vi "GVar.vi"(6 "Action":T3, 11 "Parameters In":T1={"Stop"=FALSE, "Play"=FALSE, "number of samples/ch"=12000, "sound format"={"sample rate (S/s)"=48000.0, "number of channels"=2, "bits per sample"=24}, "Path"=path ""}) -> (3 "Parameters In 2":T1={"Stop"=FALSE, "Play"=FALSE, "number of samples/ch"=12000, "sound format"={"sample rate (S/s)"=48000.0, "number of channels"=2, "bits per sample"=24}, "Path"=path ""})   [LabVIEW 2023]
uses:
  <vilib>/sound2/lvsound2.llb/Sound Data Format.ctl
  Controls/Enum 1.ctl
  Controls/Parameters In.ctl
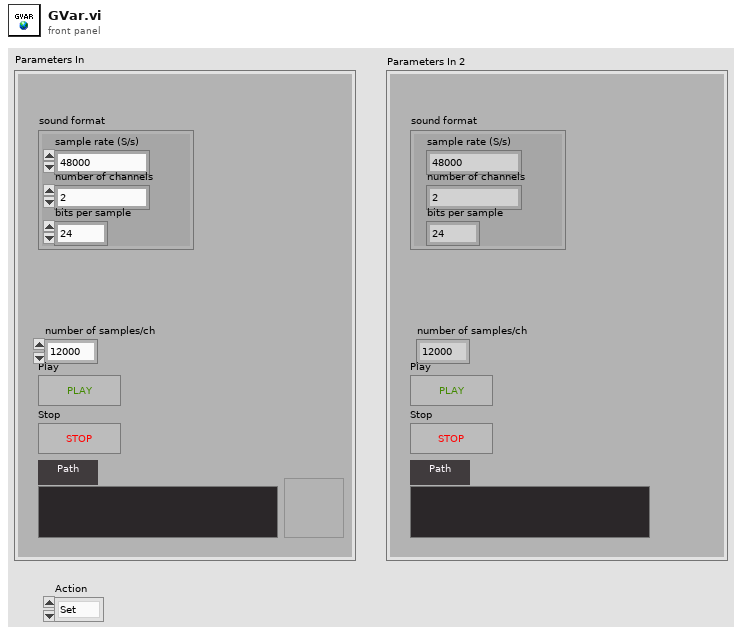
[diagram p1: front panel]
types:
  T1 = typedef "Parameters In.ctl" = cluster{"Stop":bool, "Play":bool, "number of samples/ch":i32, "sound format":T2, "Path":path}
  T2 = typedef "Sound Data Format.ctl" = cluster{"sample rate (S/s)":dbl, "number of channels":i32, "bits per sample":i32}
  T3 = typedef "Enum 1.ctl" = enum16{"Set", "Get"}
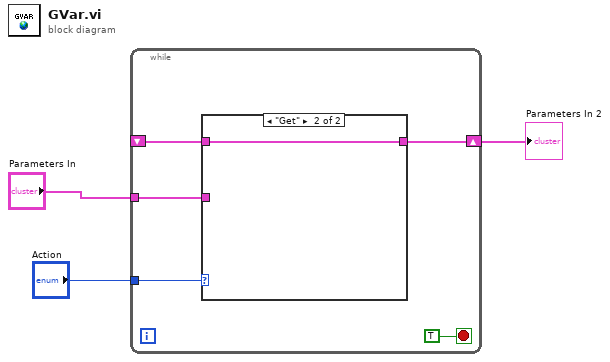
[diagram p0: block diagram]
diagram:
  n1 = while {
    shift-right: [w6] -> w1
    shift-left: _ -> [w5]
    tunnel: "Parameters In" -> [w7]
    tunnel: "Action" -> [w8]
    stop <- TRUE stop-if-true
    n2 = case shown="\"Get\"" w8 {
      tunnel: w7 -> [w9 _]
      tunnel: [w9 w10] -> w6
      tunnel: w5 -> [_ w10]
      frame "Set", Default {
      }
      frame "Get" {
      }
    }
  }
  "Parameters In 2" <- w1
